vi "runscenario Load Templates.vi"(8 "error in (no error)":errorcluster, 10 "TemplateCSV (\"\")":string, 11 "Connection Refnum":T2) -> (0 "error out":errorcluster, 2 "Templates":T1[](array[typedef]), 3 "Connection Refnum":T2)   [LabVIEW 2011]
uses:
  SI.LIB/ODBC/SQL Controls/Connection Refnum.ctl
  server/database/Templates/Template Record.ctl
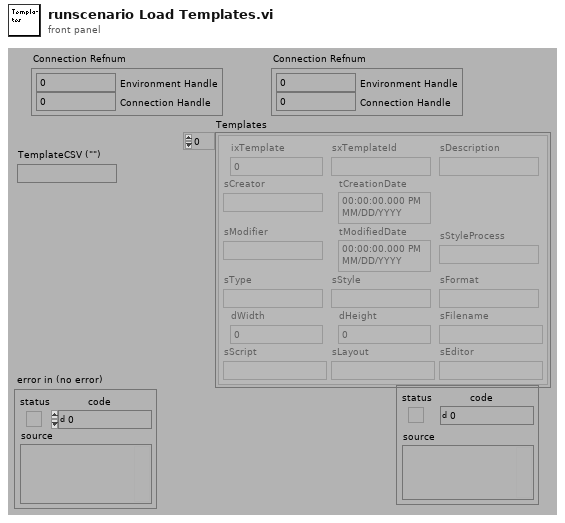
[diagram p1: front panel]
types:
  T1 = typedef "Template Record.ctl" = cluster{"ixTemplate":i32, "sxTemplateId":string, "sDescription":string, "sCreator":string, "tCreationDate":timestamp, "sModifier":string, "tModifiedDate":timestamp, "sType":string, "sStyle":string, "sFormat":string, "dWidth":dbl, "dHeight":dbl, "sFilename":string, "sScript":string, "sLayout":string, "sEditor":string, "sStyleProcess":string}
  T2 = typedef "Connection Refnum.ctl" = cluster{"Environment Handle":i32, "Connection Handle":i32}
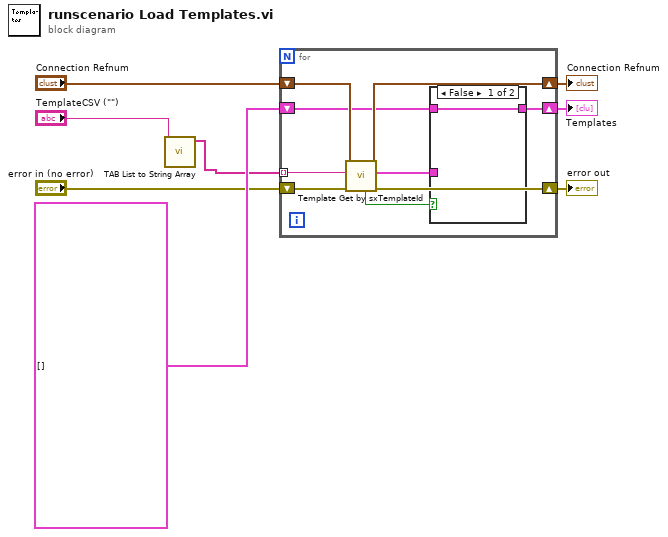
[diagram p0: block diagram]
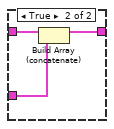
[diagram p2: hidden frame]
diagram:
  n1 = call "TAB List to String Array.vi"("String"="TemplateCSV (\"\")") -> ("Array"=w1:string[])  [unwired: 10 out]
  n2 = for {
    shift-right: [w16] -> w4
    shift-left: "error in (no error)" -> [w17]
    tunnel: w1 -> [w9] mode=indexing
    shift-right: [w14] -> w6
    shift-left: "Connection Refnum" -> [w15]
    shift-right: [w10] -> w3
    shift-left: T1[] [] -> [w12]
    n3 = call "Template Get by sxTemplateId.vi"("error in (no error)"=w17, "sxTemplateId (\"\")"=w9, "Connection Refnum"=w15) -> ("error out"=w16:errorcluster, "Template Record"=w11:T1, "Connection Refnum"=w14:T2, "Data Present"=w13:bool)  [unwired: 5 out]
    n4 = case shown="False" w13 {
      tunnel: w12 -> [w18 w21]
      tunnel: w11 -> [_ w20]
      tunnel: [w18 w19] -> w10
      frame False {
      }
      frame True {
        n5 = Build Array (concatenate)(w21, w20) -> (w19:T1[])
      }
    }
  }
  "error out" <- w4
  "Connection Refnum" <- w6
  "Templates" <- w3
